vi "AutoPickupTote.vi"() -> (2 "Done?":bool)   [LabVIEW 2014]
uses:
  Elevator/Elevator Control Command.ctl
  Elevator/Elevator Command.ctl
  Common Code/Elevator Mode.ctl
  Rollers/Roller Modes.ctl
  Common Code/Auto Roller Commands.ctl
  Common Code/Roller Mode Enum.ctl
  Common Code/Change Detect Int.vi
  Robot Global Data.vi
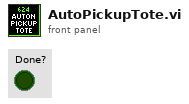
[diagram p1: front panel]
types:
  T1 = typedef "Roller Modes.ctl" = cluster{"Auto Roller Command":T2, "Roller Mode":T3}
  T2 = typedef "Auto Roller Commands.ctl" = enum16{"Grab Tote", "Idle", "Eject Tote"}
  T3 = typedef "Roller Mode Enum.ctl" = enum16{"Manual", "Safe", "Auto"}
  T4 = typedef "Elevator Control Command.ctl" = cluster{"Command":T5, "Manual Motor Out":dbl, "Manual Eject Piston":bool, "Mode":T6, "Override Limits":bool, "Manual Stabilizer":bool, "Manual Finger":bool, "Load from Step?":bool, "Store Trashcan?":bool}
  T5 = typedef "Elevator Command.ctl" = enum16{"Idle", "Load 1", "Load 2", "Load 3", "Drop Stack", "Eject Stack", "Load Trashcan"}
  T6 = typedef "Elevator Mode.ctl" = enum16{"Manual", "Safe", "Auto"}
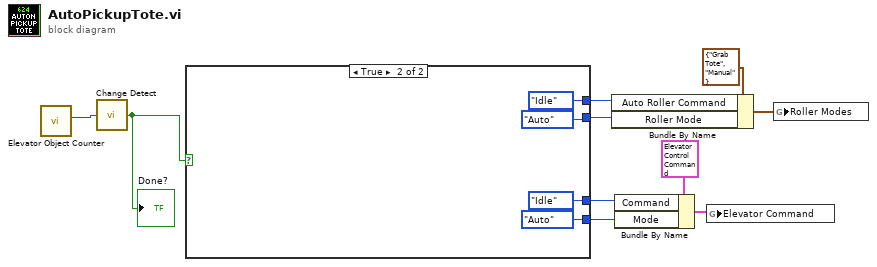
[diagram p0: block diagram]
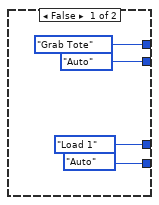
[diagram p2: hidden frame]
diagram:
  n1 = call "Elevator Object Counter.vi"() -> ("Tote Count"=w6:i8)  [unwired: 10 in, 1 out]
  n2 = call-poly "Change Detect.vi"("In"=w6) -> ("Changed?"=w5:bool)
  "Done?" <- w5
  n3 = case shown="True" w5 {
    tunnel: [Auto_Roller_Commands."Grab Tote" ("Auto Roller Command") Auto_Roller_Commands."Idle" ("Auto Roller Command")] -> w4
    tunnel: [Roller_Mode_Enum."Auto" ("Roller Mode") Roller_Mode_Enum."Auto" ("Roller Mode")] -> w3
    tunnel: [Elevator_Command."Load 1" ("Command") Elevator_Command."Idle" ("Command")] -> w2
    tunnel: [Elevator_Mode."Auto" ("Mode") Elevator_Mode."Auto" ("Mode")] -> w1
    frame False {
    }
    frame True {
    }
  }
  n4 = Bundle By Name(cluster=T1 {"Auto Roller Command"=enum."Grab Tote", "Roller Mode"=enum."Manual"} ("Roller Modes"), "Auto Roller Command"=w4, "Roller Mode"=w3) -> (w7:T1)
  n5 = Bundle By Name(cluster=T4 {"Command"=enum."Idle", "Manual Motor Out"=0.0, "Manual Eject Piston"=FALSE, "Mode"=enum."Manual", "Override Limits"=FALSE, "Manual Stabilizer"=FALSE, "Manual Finger"=FALSE, "Load from Step?"=FALSE, "Store Trashcan?"=FALSE} ("Elevator Command"), "Command"=w2, "Mode"=w1) -> (w10:T4)
  n6 = global write "Robot Global Data.vi" "Elevator Command"(w10) -> ()
  n7 = global write "Robot Global Data.vi" "Roller Modes"(w7) -> ()
